vi "Quaternion_Inverse.vi"(11 "Quaternion":T1={"R"=1.0, "V"=[0.0, 0.0, 0.0]}) -> (3 "Inverse":T1={"R"=1.0, "V"=[0.0, 0.0, 0.0]})   [LabVIEW 2019, in "Trajectory_Library.lvlib"]
doc: "Returns the inverse of the quaternion.\nParameters:\n - Quaternion - Quaternion data cluster\n\nReturns:\n - Inverse - The inverse quaternion data cluster."
uses:
  Trajectory_Library.lvlib
  TypeDef/QUATERNION.ctl
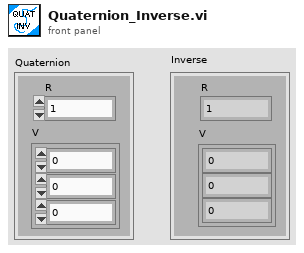
[diagram p1: front panel]
types:
  T1 = typedef "Trajectory_Library.lvlib/QUATERNION.ctl" = cluster{"R":dbl, "V":dbl[]}
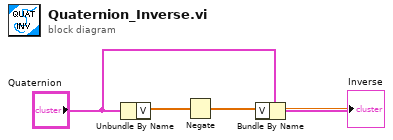
[diagram p0: block diagram]
diagram:
  n1 = Unbundle By Name("Quaternion") -> ("V"=w2:dbl[])
  n2 = Negate(x=w2) -> (-x=w1:dbl[])
  n3 = Bundle By Name(cluster="Quaternion", "V"=w1) -> (→"Inverse":T1)
